vi "PID_Controller_Interface.vi"() -> ()   [LabVIEW 2019]
uses:
  <vilib>/Instr/_visa.llb/VISA Open Access Mode.ctl
  <vilib>/Instr/_visa.llb/VISA Flush IO Buffer Mask.ctl
  <vilib>/Instr/_visa.llb/VISA Configure Serial Port (Instr).vi
panel:
  out "ms":i32
  out "temp":dbl
  in  "readbuffer2clear":bool
  out "read buffer 2":string
  in  "Ts":dbl=1.0
  out "read buffer":string
  in  "COMError":errorcluster
  in  "Setpoint":bool
  in  "Temperature Setpoint":dbl=35.0
  in  "Stop":bool
  in  "Run":bool
  out "COMStatus":bool
  in  "SetConnection":bool
  in  "COM Port":refnum<visa-resource-name>
  in  "SetPIDParams":bool
  in  "Kd":dbl=1.0
  in  "Ki":dbl=1.0
  in  "Kp":dbl=1.0
  out "Waveform Chart":dbl(graph)
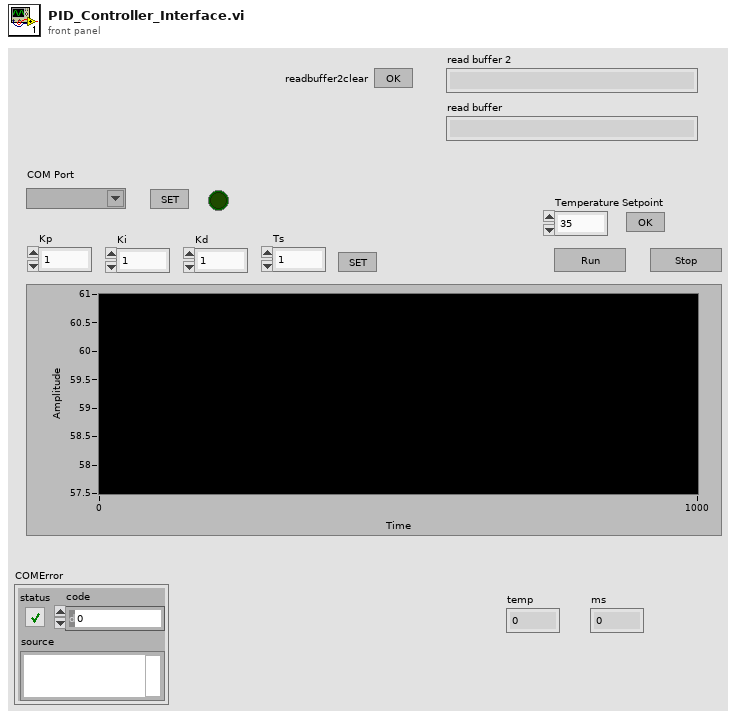
[diagram p1: front panel]
types:
  T1 = typedef "VISA Flush IO Buffer Mask.ctl" = u16
  T2 = typedef "VISA Open Access Mode.ctl" = u32
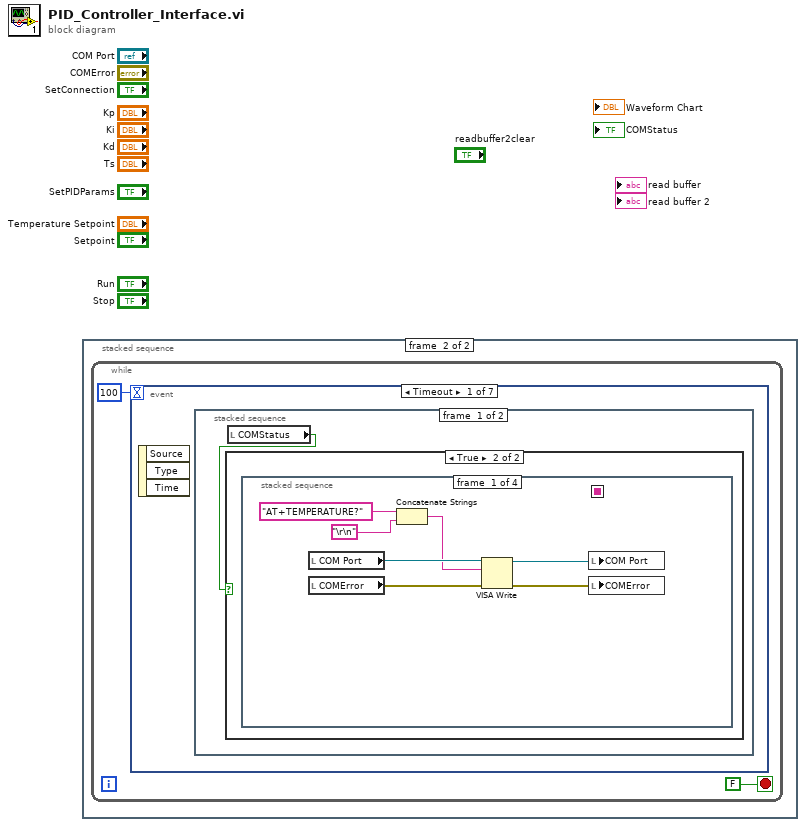
[diagram p0: block diagram]
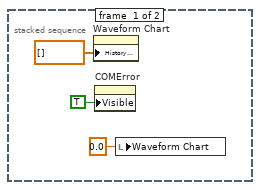
[diagram p2: hidden frame]
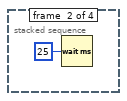
[diagram p4: hidden frame]
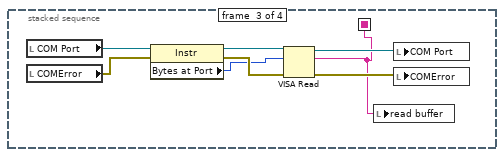
[diagram p5: hidden frame]
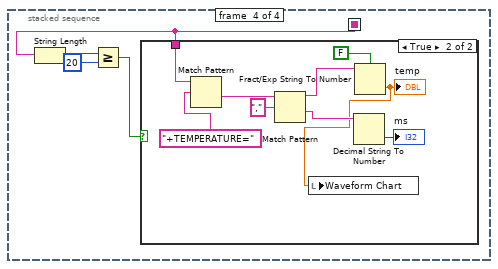
[diagram p6: hidden frame]
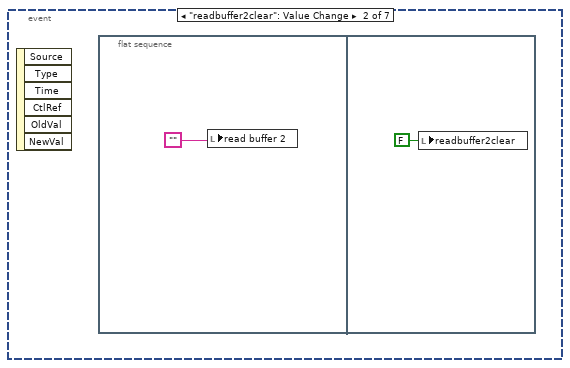
[diagram p9: hidden frame]
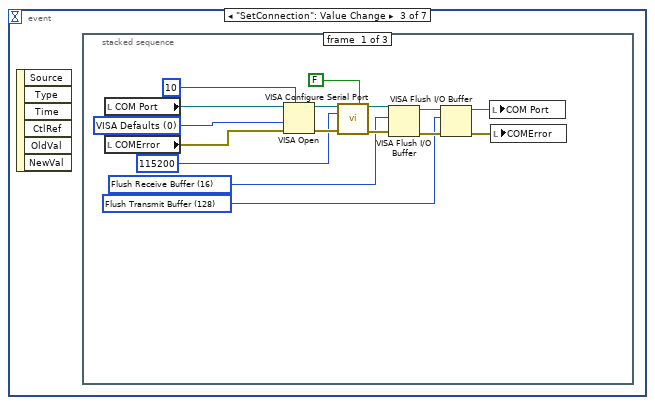
[diagram p10: hidden frame]
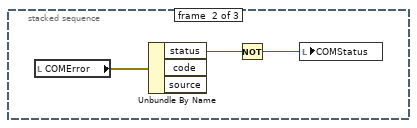
[diagram p11: hidden frame]
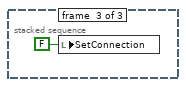
[diagram p12: hidden frame]
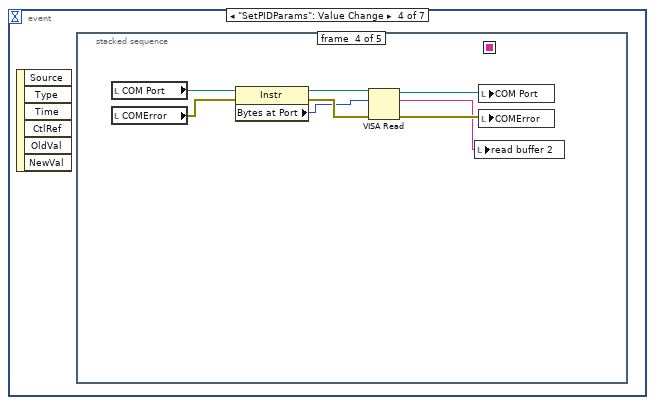
[diagram p13: hidden frame]
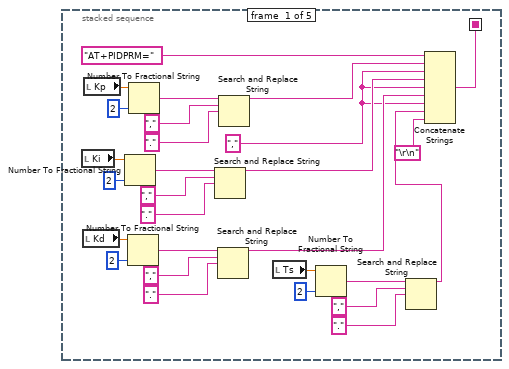
[diagram p14: hidden frame]
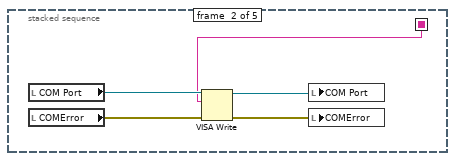
[diagram p15: hidden frame]
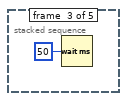
[diagram p16: hidden frame]
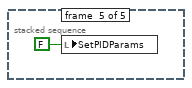
[diagram p17: hidden frame]
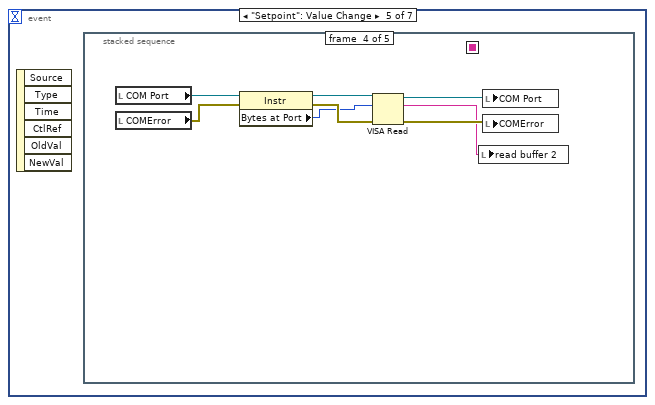
[diagram p18: hidden frame]
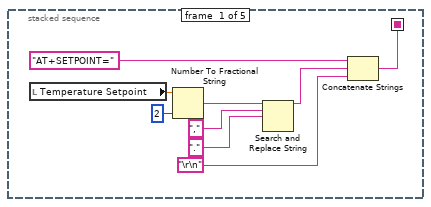
[diagram p19: hidden frame]
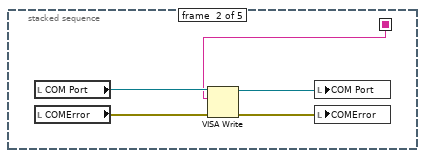
[diagram p20: hidden frame]
diagram:
  n1 = stacked-sequence {
    frame #0 {
      n2 = property on="Waveform Chart" class="WFChart (strict)"("History Data"=dbl[] []) -> ()  [unwired: 2 in, 2 out]
      n3 = property on="COMError" class="Clust (strict)"("Visible"=TRUE) -> ()  [unwired: 2 in, 2 out]
      n4 = local write "Waveform Chart"(0.0 ("Waveform Chart")) -> ()
    }
    frame #1 {
      n5 = while {
        stop <- FALSE stop-if-true
        n6 = event shown="[0] Timeout" {
          selector: _ -> [_ _ _ _ _ _ _]
          dyn-events: _ -> [_ _ _ _ _ _ _]
          timeout: 100 -> [_ _ _ _ _ _ _]
          event Timeout {
            n7 = event-data() -> ()  [unwired: 1 in, 3 out]
            n8 = stacked-sequence {
              frame #0 {
                n9 = local read "COMStatus"() -> (w6:bool)
                n10 = case shown="True" w6 {
                  frame False {
                  }
                  frame True {
                    n11 = stacked-sequence {
                      seq-local: [_ _ w15 _] -> [_ _ _ w23]
                      frame #0 {
                        n12 = local read "COM Port"() -> (w11:refnum<visa-resource-name>)
                        n13 = local read "COMError"() -> (w9:errorcluster)
                        n14 = Concatenate Strings("AT+TEMPERATURE?", "\r\n") -> (w7:string)
                        n15 = VISA Write(VISA resource name=w11, write buffer=w7, error in (no error)=w9) -> (VISA resource name out=w10:refnum<visa-resource-name>, error out=w8:errorcluster)  [unwired: 1 out]
                        n16 = local write "COM Port"(w10) -> ()
                        n17 = local write "COMError"(w8) -> ()
                      }
                      frame #1 {
                        n18 = Wait (ms)(milliseconds to wait=u32 25) -> ()  [unwired: 1 out]
                      }
                      frame #2 {
                        n19 = local read "COM Port"() -> (w22:refnum<visa-resource-name>)
                        n20 = local read "COMError"() -> (w21:errorcluster)
                        n21 = property class="Instr"(reference=w22, error in=w21) -> (reference out=w20:refnum<visa-resource-name>, error out=w19:errorcluster, "Bytes at Port"=w18:u32)
                        n22 = VISA Read(VISA resource name=w20, byte count=w18, error in (no error)=w19) -> (VISA resource name out=w17:refnum<visa-resource-name>, read buffer=w15:string, error out=w16:errorcluster)  [unwired: 1 out]
                        n23 = local write "read buffer"(w15) -> ()
                        n24 = local write "COM Port"(w17) -> ()
                        n25 = local write "COMError"(w16) -> ()
                      }
                      frame #3 {
                        n26 = String Length(string=w23) -> (length=w26:i32)
                        n27 = Greater Or Equal?(x=w26, y=20) -> (x >= y?=w24:bool)
                        n28 = case shown="True" w24 {
                          tunnel: w23 -> [_ w35]
                          frame False {
                          }
                          frame True {
                            n29 = Match Pattern(string=w35, regular expression="+TEMPERATURE=") -> (after substring=w33:string)  [unwired: 1 in, 3 out]
                            n30 = Match Pattern(string=w33, regular expression=",") -> (before substring=w31:string, after substring=w30:string)  [unwired: 1 in, 2 out]
                            n31 = Decimal String To Number(string=w30) -> (number=→"ms":i32)  [unwired: 2 in, 1 out]
                            n32 = Fract/Exp String To Number(use system decimal point (T)=FALSE, string=w31) -> (number=w27:dbl)  [unwired: 2 in, 1 out]
                            "temp" <- w27
                            n33 = local write "Waveform Chart"(w27) -> ()
                          }
                        }
                      }
                    }
                  }
                }
              }
              frame #1 {
              }
            }
          }
          event "readbuffer2clear": Value Change {
            n34 = event-data() -> ()  [unwired: 1 in, 6 out]
            n35 = flat-sequence {
              frame #0 {
                n36 = local write "read buffer 2"("") -> ()
              }
              frame #1 {
                n37 = local write "readbuffer2clear"(FALSE ("readbuffer2clear")) -> ()
              }
            }
          }
          event "SetConnection": Value Change {
            n38 = event-data() -> ()  [unwired: 1 in, 6 out]
            n39 = stacked-sequence {
              frame #0 {
                w40 = T1 128 items=["Flush Receive Buffer"=16, "Write Transmit Buffer to Device"=32, "Flush Receive Buffer (No I/O)"=64, "Flush Transmit Buffer"=128] ("Mask")
                w43 = T1 16 items=["Flush Receive Buffer"=16, "Write Transmit Buffer to Device"=32, "Flush Receive Buffer (No I/O)"=64, "Flush Transmit Buffer"=128] ("Mask")
                w52 = T2 0 items=["VISA Defaults"=0, "Exclusive Lock"=1, "Load Configured Settings"=4] ("Access Mode")
                n40 = local read "COM Port"() -> (w53:refnum<visa-resource-name>)
                n41 = local read "COMError"() -> (w51:errorcluster)
                n42 = VISA Open(timeout (0)=u32 10 ("VISA Open timeout (0)"), access mode=w52, error in (no error)=w51, VISA resource name=w53) -> (VISA resource name=w49:refnum<visa-resource-name>, error out=w48:errorcluster)  [unwired: 1 in]
                n43 = call-poly "VISA Configure Serial Port"("VISA resource name"=w49, "Enable Termination\nChar (T)"=FALSE ("Enable Termination\nChar (T)"), "baud rate (9600)"=u32 115200, "error in (no error)"=w48) -> ("VISA resource name out"=w45:refnum<visa-resource-name>, "error out"=w44:errorcluster)  [unwired: 10 in]
                n44 = VISA Flush I/O Buffer(VISA resource name=w45, mask (16)=w43, error in (no error)=w44) -> (VISA resource name out=w42:refnum<visa-resource-name>, error out=w41:errorcluster)
                n45 = VISA Flush I/O Buffer(VISA resource name=w42, mask (16)=w40, error in (no error)=w41) -> (VISA resource name out=w39:refnum<visa-resource-name>, error out=w38:errorcluster)
                n46 = local write "COM Port"(w39) -> ()
                n47 = local write "COMError"(w38) -> ()
              }
              frame #1 {
                n48 = local read "COMError"() -> (w56:errorcluster)
                n49 = Unbundle By Name(w56) -> ("status"=w55:bool)  [unwired: 2 out]
                n50 = Not(x=w55) -> (.not. x?=w54:bool)
                n51 = local write "COMStatus"(w54) -> ()
              }
              frame #2 {
                n52 = local write "SetConnection"(FALSE ("SetConnection")) -> ()
              }
            }
          }
          event "SetPIDParams": Value Change {
            n53 = event-data() -> ()  [unwired: 1 in, 6 out]
            n54 = stacked-sequence {
              seq-local: [w61 _ _ _ _] -> [_ w86 _ _ _]
              frame #0 {
                w58 = ","
                n55 = local read "Ki"() -> (w74:dbl)
                n56 = local read "Kd"() -> (w73:dbl)
                n57 = local read "Kp"() -> (w85:dbl)
                n58 = Number To Fractional String(number=w74, precision (6)=i16 2) -> (F-format string=w75:string)  [unwired: 2 in]
                n59 = Number To Fractional String(number=w73, precision (6)=i16 2) -> (F-format string=w72:string)  [unwired: 2 in]
                n60 = Number To Fractional String(number=w85, precision (6)=i16 2) -> (F-format string=w84:string)  [unwired: 2 in]
                n61 = Search and Replace String(input string=w75, search string=",", replace string="." ("replace string (\"\")")) -> (result string=w68:string)  [unwired: 5 in, 3 out]
                n62 = Search and Replace String(input string=w72, search string=",", replace string="." ("replace string (\"\")")) -> (result string=w67:string)  [unwired: 5 in, 3 out]
                n63 = Search and Replace String(input string=w84, search string=",", replace string="." ("replace string (\"\")")) -> (result string=w83:string)  [unwired: 5 in, 3 out]
                n64 = local read "Ts"() -> (w62:dbl)
                n65 = Number To Fractional String(number=w62, precision (6)=i16 2) -> (F-format string=w63:string)  [unwired: 2 in]
                n66 = Search and Replace String(input string=w63, search string=",", replace string="." ("replace string (\"\")")) -> (result string=w59:string)  [unwired: 5 in, 3 out]
                n67 = Concatenate Strings("AT+PIDPRM=", w83, w58, w68, w58, w67, w58, w59, "\r\n") -> (w61:string)
              }
              frame #1 {
                n68 = local read "COM Port"() -> (w90:refnum<visa-resource-name>)
                n69 = local read "COMError"() -> (w88:errorcluster)
                n70 = VISA Write(VISA resource name=w90, write buffer=w86, error in (no error)=w88) -> (VISA resource name out=w89:refnum<visa-resource-name>, error out=w87:errorcluster)  [unwired: 1 out]
                n71 = local write "COM Port"(w89) -> ()
                n72 = local write "COMError"(w87) -> ()
              }
              frame #2 {
                n73 = Wait (ms)(milliseconds to wait=u32 50) -> ()  [unwired: 1 out]
              }
              frame #3 {
                n74 = local read "COM Port"() -> (w99:refnum<visa-resource-name>)
                n75 = local read "COMError"() -> (w98:errorcluster)
                n76 = property class="Instr"(reference=w99, error in=w98) -> (reference out=w97:refnum<visa-resource-name>, error out=w96:errorcluster, "Bytes at Port"=w95:u32)
                n77 = VISA Read(VISA resource name=w97, byte count=w95, error in (no error)=w96) -> (VISA resource name out=w94:refnum<visa-resource-name>, read buffer=w92:string, error out=w93:errorcluster)  [unwired: 1 out]
                n78 = local write "read buffer 2"(w92) -> ()
                n79 = local write "COM Port"(w94) -> ()
                n80 = local write "COMError"(w93) -> ()
              }
              frame #4 {
                n81 = local write "SetPIDParams"(FALSE ("SetConnection")) -> ()
              }
            }
          }
          event "Setpoint": Value Change {
            n82 = event-data() -> ()  [unwired: 1 in, 6 out]
            n83 = stacked-sequence {
              seq-local: [w101 _ _ _ _] -> [_ w110 _ _ _]
              frame #0 {
                n84 = local read "Temperature Setpoint"() -> (w109:dbl)
                n85 = Number To Fractional String(number=w109, precision (6)=i16 2) -> (F-format string=w106:string)  [unwired: 2 in]
                n86 = Search and Replace String(input string=w106, search string=",", replace string="." ("replace string (\"\")")) -> (result string=w103:string)  [unwired: 5 in, 3 out]
                n87 = Concatenate Strings("AT+SETPOINT=", w103, "\r\n") -> (w101:string)
              }
              frame #1 {
                n88 = local read "COM Port"() -> (w114:refnum<visa-resource-name>)
                n89 = local read "COMError"() -> (w112:errorcluster)
                n90 = VISA Write(VISA resource name=w114, write buffer=w110, error in (no error)=w112) -> (VISA resource name out=w113:refnum<visa-resource-name>, error out=w111:errorcluster)  [unwired: 1 out]
                n91 = local write "COM Port"(w113) -> ()
                n92 = local write "COMError"(w111) -> ()
              }
              frame #2 {
                n93 = Wait (ms)(milliseconds to wait=u32 50) -> ()  [unwired: 1 out]
              }
              frame #3 {
                n94 = local read "COM Port"() -> (w123:refnum<visa-resource-name>)
                n95 = local read "COMError"() -> (w122:errorcluster)
                n96 = property class="Instr"(reference=w123, error in=w122) -> (reference out=w121:refnum<visa-resource-name>, error out=w120:errorcluster, "Bytes at Port"=w119:u32)
                n97 = VISA Read(VISA resource name=w121, byte count=w119, error in (no error)=w120) -> (VISA resource name out=w118:refnum<visa-resource-name>, read buffer=w116:string, error out=w117:errorcluster)  [unwired: 1 out]
                n98 = local write "read buffer 2"(w116) -> ()
                n99 = local write "COM Port"(w118) -> ()
                n100 = local write "COMError"(w117) -> ()
              }
              frame #4 {
                n101 = local write "Setpoint"(FALSE ("SetConnection")) -> ()
              }
            }
          }
          event "Run": Value Change {
            n102 = event-data() -> ()  [unwired: 1 in, 6 out]
            n103 = stacked-sequence {
              seq-local: [w125 _ _ _ _] -> [_ w128 _ _ _]
              frame #0 {
                n104 = Concatenate Strings("AT+CONTROL=1", "\r\n") -> (w125:string)
              }
              frame #1 {
                n105 = local read "COM Port"() -> (w132:refnum<visa-resource-name>)
                n106 = local read "COMError"() -> (w130:errorcluster)
                n107 = VISA Write(VISA resource name=w132, write buffer=w128, error in (no error)=w130) -> (VISA resource name out=w131:refnum<visa-resource-name>, error out=w129:errorcluster)  [unwired: 1 out]
                n108 = local write "COM Port"(w131) -> ()
                n109 = local write "COMError"(w129) -> ()
              }
              frame #2 {
                n110 = Wait (ms)(milliseconds to wait=u32 50) -> ()  [unwired: 1 out]
              }
              frame #3 {
                n111 = local read "COM Port"() -> (w141:refnum<visa-resource-name>)
                n112 = local read "COMError"() -> (w140:errorcluster)
                n113 = property class="Instr"(reference=w141, error in=w140) -> (reference out=w139:refnum<visa-resource-name>, error out=w138:errorcluster, "Bytes at Port"=w137:u32)
                n114 = VISA Read(VISA resource name=w139, byte count=w137, error in (no error)=w138) -> (VISA resource name out=w136:refnum<visa-resource-name>, read buffer=w134:string, error out=w135:errorcluster)  [unwired: 1 out]
                n115 = local write "read buffer 2"(w134) -> ()
                n116 = local write "COM Port"(w136) -> ()
                n117 = local write "COMError"(w135) -> ()
              }
              frame #4 {
                n118 = local write "Run"(FALSE ("SetConnection")) -> ()
              }
            }
          }
          event "Stop": Value Change {
            n119 = event-data() -> ()  [unwired: 1 in, 6 out]
            n120 = stacked-sequence {
              seq-local: [w143 _ _ _ _] -> [_ w146 _ _ _]
              frame #0 {
                n121 = Concatenate Strings("AT+CONTROL=0", "\r\n") -> (w143:string)
              }
              frame #1 {
                n122 = local read "COM Port"() -> (w150:refnum<visa-resource-name>)
                n123 = local read "COMError"() -> (w148:errorcluster)
                n124 = VISA Write(VISA resource name=w150, write buffer=w146, error in (no error)=w148) -> (VISA resource name out=w149:refnum<visa-resource-name>, error out=w147:errorcluster)  [unwired: 1 out]
                n125 = local write "COM Port"(w149) -> ()
                n126 = local write "COMError"(w147) -> ()
              }
              frame #2 {
                n127 = Wait (ms)(milliseconds to wait=u32 50) -> ()  [unwired: 1 out]
              }
              frame #3 {
                n128 = local read "COM Port"() -> (w159:refnum<visa-resource-name>)
                n129 = local read "COMError"() -> (w158:errorcluster)
                n130 = property class="Instr"(reference=w159, error in=w158) -> (reference out=w157:refnum<visa-resource-name>, error out=w156:errorcluster, "Bytes at Port"=w155:u32)
                n131 = VISA Read(VISA resource name=w157, byte count=w155, error in (no error)=w156) -> (VISA resource name out=w154:refnum<visa-resource-name>, read buffer=w152:string, error out=w153:errorcluster)  [unwired: 1 out]
                n132 = local write "read buffer 2"(w152) -> ()
                n133 = local write "COM Port"(w154) -> ()
                n134 = local write "COMError"(w153) -> ()
              }
              frame #4 {
                n135 = local write "Stop"(FALSE ("SetConnection")) -> ()
              }
            }
          }
        }
      }
    }
  }
